vi "Read Style.vi"(8 "error in (no error)":errorcluster, 11 "PathCommands in":refnum<class "PathCommands.lvclass">) -> (0 "error out":errorcluster, 2 "CSSProperties.lvclass":refnum<class "CSSProperties.lvclass">, 3 "PathCommands out":refnum<class "PathCommands.lvclass">)   [LabVIEW 2020]
uses:
  PathCommands.lvclass
  CSSProperties/CSSProperties.lvclass
  PathCommands.lvclass/PathCommands.ctl
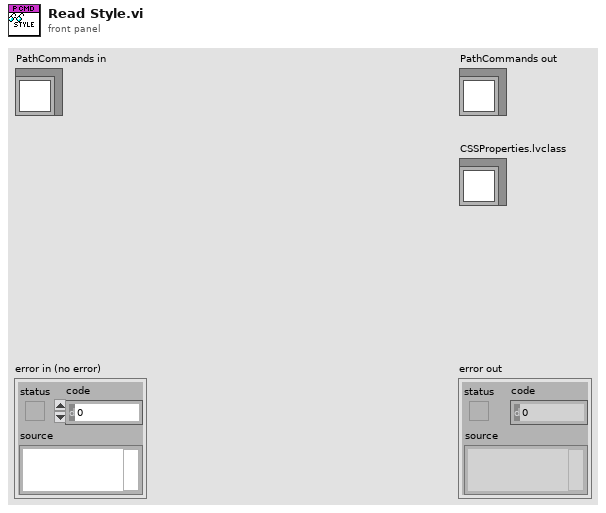
[diagram p1: front panel]
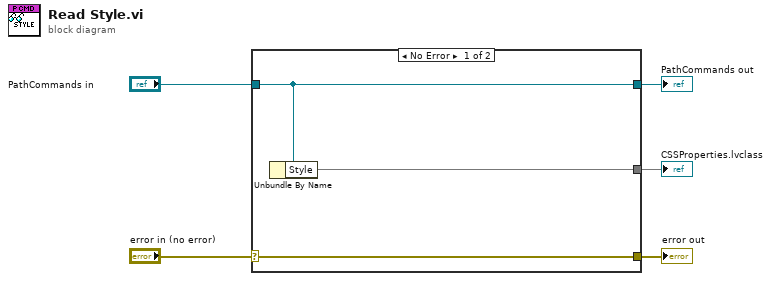
[diagram p0: block diagram]
diagram:
  n1 = case shown="No Error" "error in (no error)" {
    selector: "error in (no error)" -> [w8 w9]
    tunnel: [w8 w9] -> w4
    tunnel: [w7 w10] -> w2
    tunnel: "PathCommands in" -> [w7 w10]
    tunnel: [w6 _] -> w1
    frame No Error {
      n2 = Unbundle By Name(w7) -> ("Style"=w6)
    }
    frame Error {
    }
  }
  "error out" <- w4
  "PathCommands out" <- w2
  "CSSProperties.lvclass" <- w1
